vi "From String Cluster.vi"(0 "Pair":cluster{"Key":string, "Value":string}) -> (2 "Map":refnum<class "Map.lvclass">)   [LabVIEW 2018, in "Toolkit.lvlib" / "Data.lvlib" / "Map.lvclass"]
uses:
  Map.lvclass
  Map.lvclass/Map.ctl
  String/String.lvclass
  D:/Users/cfield/Code/Field R&D Services/Mustache/LabVIEW/trunk/src/Toolkit/Data/Datum/Datum.lvclass
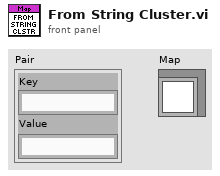
[diagram p1: front panel]
types:
  T1 = cluster{"Key":string, "String":refnum<class "String.lvclass">}
  T2 = cluster{"Key":string, "String":refnum<class "String.lvclass">}[]
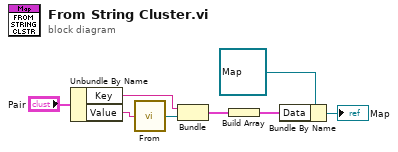
[diagram p0: block diagram]
diagram:
  n1 = Unbundle By Name("Pair") -> ("Key"=w3:string, "Value"=w4:string)
  n2 = call "From.vi"("Value"=w4) -> ("String"=w2:refnum<class "String.lvclass">)
  n3 = Bundle("Key"=w3, "String"=w2) -> (w1:T1)  [unwired: 1 in]
  n4 = Build Array(w1) -> (w6:T2)
  n5 = Bundle By Name(cluster=refnum<class "Map.lvclass"> refnum ("Toolkit.lvlib:Data.lvlib:Map.lvclass"), "Data"=w6) -> (→"Map":refnum<class "Map.lvclass">)
